vi "polar_test_ciz.vi"() -> ()   [LabVIEW 2016]
uses:
  <vilib>/silver_ctls/ArrayMatrixCluster/Real Matrix NI_Silver.ctl
panel:
  in  "Teta":i32
  in  "polar attributes":T1={"maximum"=0.0, "minimum"=0.0, "clip to min"=FALSE, "log?(F)"=FALSE, "grid color"=6710886, "plot color"=16711680, "fmt and prec"={"format"=enum."Decimal", "precision"=0}, "visible section"=8} {"minimum" format="%0.2f"; "maximum" format="%0.2f"}
  out "XY Graph 2":cluster{i32[], "Real Matrix":dbl[]}(graph)
  out "Polar Plot":picture
  out "Array1":dbl[](array[numeric])
  out "Real Matrix":T2
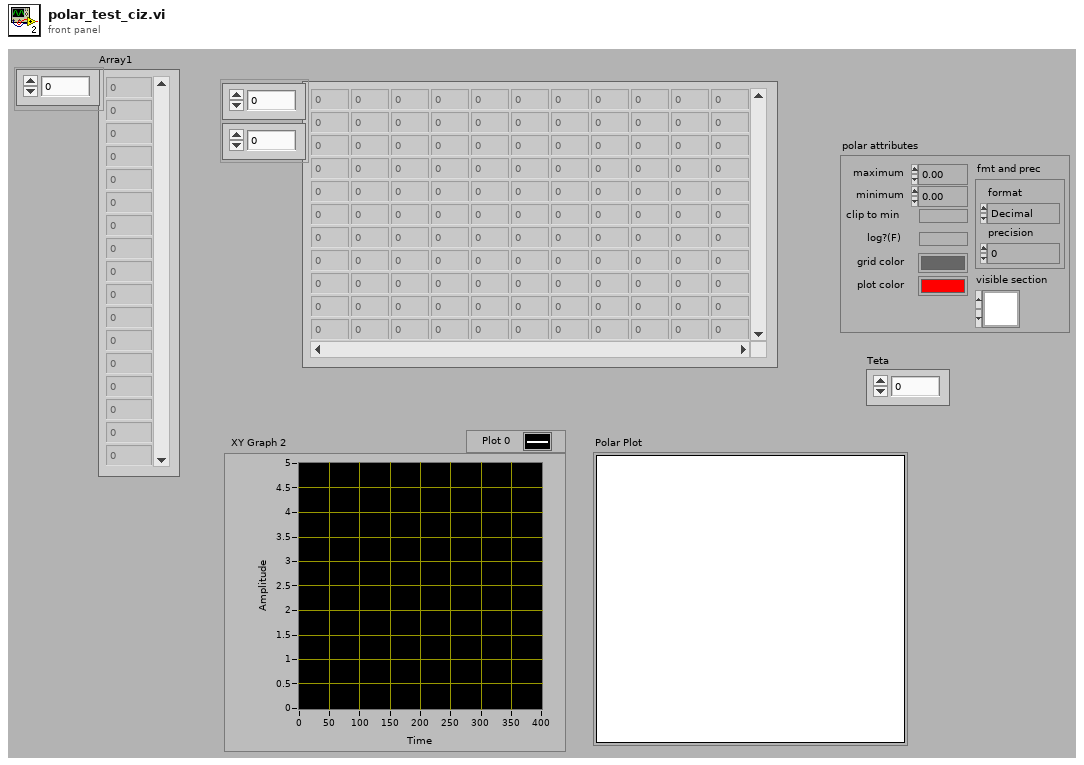
[diagram p1: front panel]
types:
  T1 = cluster{"maximum":dbl, "minimum":dbl, "clip to min":bool, "log?(F)":bool, "grid color":u32, "plot color":u32, "fmt and prec":cluster{"format":enum8{"Decimal", "Scientific", "Engineering", "Binary", "Octal", "Hex"}, "precision":u8}, "visible section":u16}
  T2 = typedef "Real Matrix NI_Silver.ctl" = dbl[][]
  T3 = typedef "NI_Matrix.lvlib/RealMatrix.ctl" = dbl[][]
  T4 = typedef "LVBoundsTypeDef.ctl" = cluster{"Width":u32, "Height":u32}
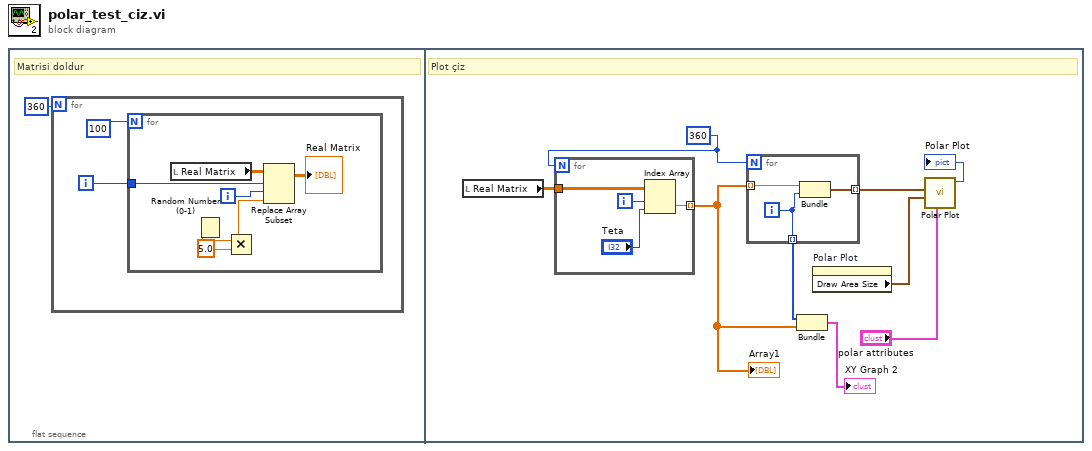
[diagram p0: block diagram]
diagram:
  n1 = flat-sequence {
    frame #0 {
      # "Matrisi doldur"
      n2 = for {
        N: 360 -> [_]
        i -> [w3]
        n3 = for {
          N: 100 -> [_]
          tunnel: w3 -> [w5]
          i -> [w4]
          n4 = local read "Real Matrix"() -> (w10:T2)
          n5 = Random Number (0-1)() -> (number: 0 to 1=w7:dbl)
          n6 = Multiply(x=w7, y=5.0) -> (x*y=w6:dbl)
          n7 = Replace Array Subset ("Set Matrix Elements")(array=w10, new element=w6, index (row)=w5, index (col)=w4) -> (→"Real Matrix":T3)
        }
      }
    }
    frame #1 {
      w11 = 360
      # "Plot çiz"
      n8 = local read "Real Matrix"() -> (w14:T2)
      n9 = for {
        N: w11 -> [_]
        tunnel: [w26] -> w12 mode=indexing
        tunnel: w14 -> [w25]
        i -> [w24]
        n10 = Index Array(array=w25, index (row)=w24, index (col)="Teta") -> (element=w26:dbl)
      }
      "Array1" <- w12
      n11 = for {
        N: w11 -> [_]
        tunnel: [w21] -> w16 mode=indexing
        tunnel: w12 -> [w22] mode=indexing
        tunnel: [w20] -> w13 mode=indexing
        i -> [w20]
        n12 = Bundle("Numeric"=w22, w20) -> (w21:cluster{"Numeric":dbl, i32})  [unwired: 1 in]
      }
      n13 = Bundle(w13, w12) -> (→"XY Graph 2":cluster{i32[], dbl[]})  [unwired: 1 in]
      n14 = property on="Polar Plot" class="Pict"() -> ("Draw Area Size"=w17:T4)  [unwired: 2 in, 2 out]
      n15 = call <vilib>:"Polar Plot.vi"("polar attributes"="polar attributes", "dimensions (w,h)"=w17, "data array [mag, phase (deg)]"=w16) -> ("new picture"=→"Polar Plot":picture)  [unwired: 8 in]
    }
  }
